vi "动作检查.vi"(8 "无误":errorcluster caption="错误输入", 9 "需要动作":string, 10 "动作枚举类型匹配?":bool, 11 "传入动作":string) -> (0 "输出簇":errorcluster caption="错误输出")   [LabVIEW 2017, in "模块模板.lvlib"]
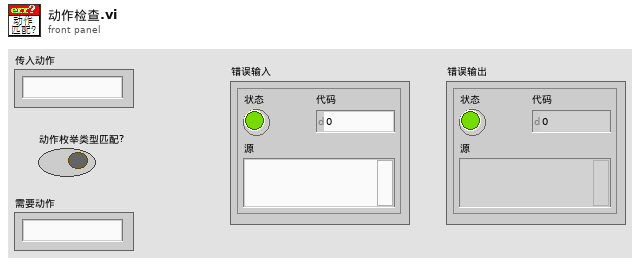
[diagram p1: front panel]
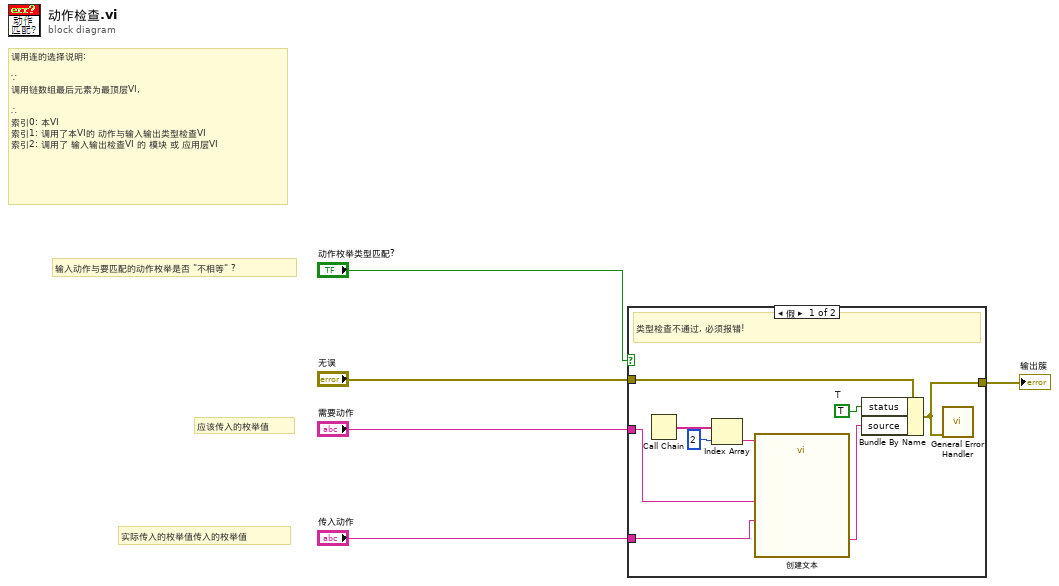
[diagram p0: block diagram]
diagram:
  # "实际传入的枚举值传入的枚举值"
  # "应该传入的枚举值"
  # "输入动作与要匹配的动作枚举是否 \"不相等\" ?"
  # "调用连的选择说明:\n\n∵ \n调用链数组最后元素为最顶层VI,\n\n∴ \n索引0: 本VI\n索引1: 调用了本VI的 动作与输入输出类型检查VI\n索引2: 调用了 输入输出检查VI 的 模块 或 应用层VI"
  n1 = case shown="假" "动作枚举类型匹配?" {
    tunnel: "需要动作" -> [w11 _]
    tunnel: "传入动作" -> [w10 _]
    tunnel: [w7 w15] -> w2
    tunnel: "无误" -> [w6 w15]
    frame False {
      w8 = TRUE  # T
      # "类型检查不通过, 必须报错!"
      n2 = Call Chain() -> (call chain=w13:string[])
      n3 = Index Array(array=w13, index=2 ("索引")) -> (element=w12:string)
      n4 = call "创建文本"("Beginning Text"=w12, "需要动作"=w11, "传入动作"=w10) -> ("Result"=w14:string)  [unwired: 11 in, 1 out]
      n5 = Bundle By Name(cluster=w6, "status"=w8, "source"=w14) -> (w7:errorcluster)
      n6 = call <vilib>:"General Error Handler.vi"("error in (no error)"=w7) -> ()  [unwired: 10 in, 5 out]
    }
    frame True {
    }
  }
  "输出簇" <- w2
